vi "MotorInit.vi"(2 "错误输入":errorcluster) -> (0 "错误输出":errorcluster, 1 "通信成功？":bool)   [LabVIEW 2018]
panel:
  out "网卡":string[](array[string])
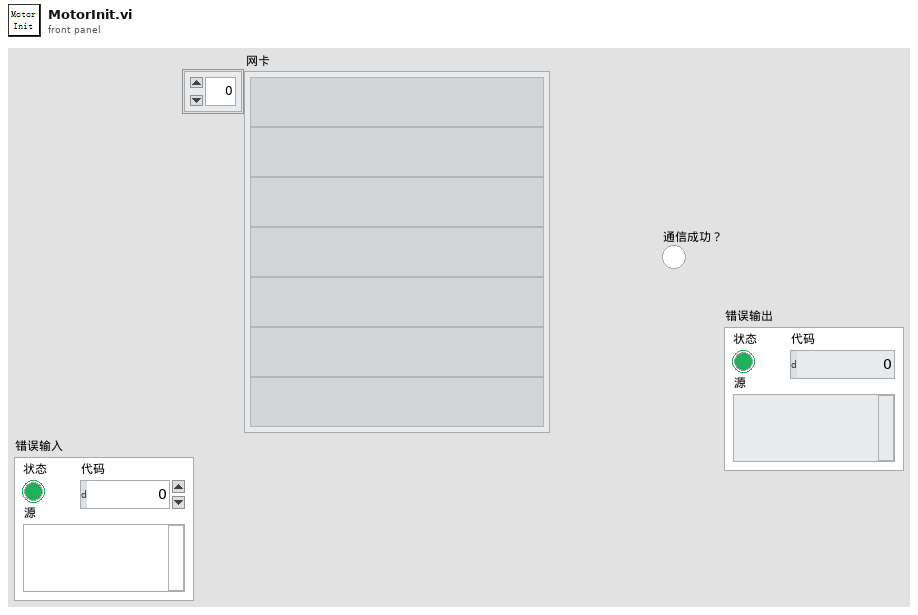
[diagram p1: front panel]
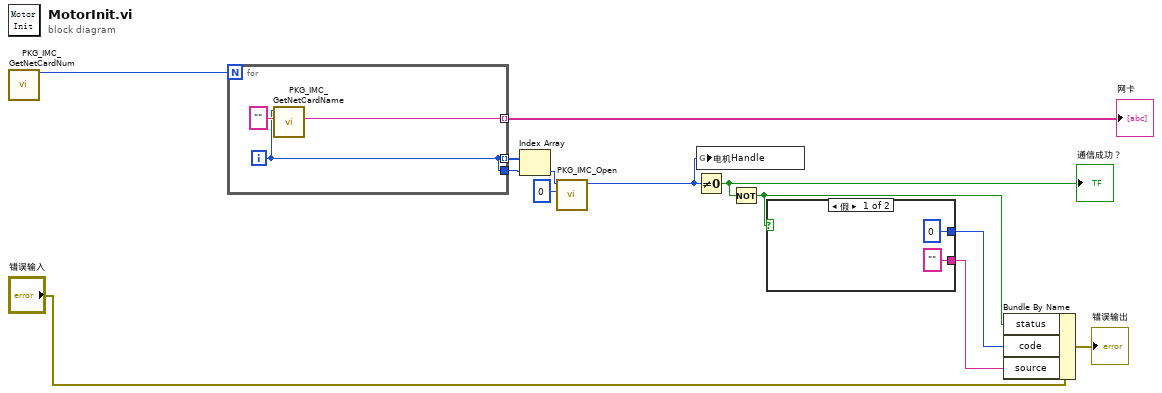
[diagram p0: block diagram]
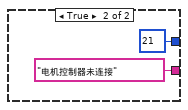
[diagram p2: hidden frame]
diagram:
  n1 = call "PKG_IMC_GetNetCardNum.vi"() -> ("function return"=w13:i32)  [unwired: 11 in]
  n2 = for {
    N: w13 -> [_]
    tunnel: [w15] -> w9 mode=indexing
    tunnel: [w14] -> w12 mode=indexing
    tunnel: [w14] -> w7
    i -> [w14]
    n3 = call "PKG_IMC_GetNetCardName.vi"("name"="", "index"=w14) -> ("name out"=w15:string)  [unwired: 8 in, 1 out]
  }
  "网卡" <- w9
  n4 = Index Array(array=w12, index=w7) -> (element=w11:i32)
  n5 = call "PKG_IMC_Open.vi"("imcid"=0, "netcardsel"=w11) -> ("function return"=w8:u32)  [unwired: 9 in]
  n6 = Not Equal To 0?(x=w8) -> (x != 0?=w5:bool)
  "通信成功？" <- w5
  n7 = global write "参数.vi" "电机Handle"(w8) -> ()
  n8 = Not(x=w5) -> (.not. x?=w4:bool)
  n9 = case shown="假" w4 {
    tunnel: ["" "电机控制器未连接" ("source")] -> w3
    tunnel: [0 ("code") 21 ("code")] -> w1
    frame False {
    }
    frame True {
    }
  }
  n10 = Bundle By Name(cluster="错误输入", "status"=w4, "code"=w1, "source"=w3) -> (→"错误输出":errorcluster)
